vi "F-Zones.vi"(8 "Filter Prams In":T3, 10 "Trans Geometry (mm)":T1={"Transducer"=0, "Geo Focus"=12.0, "a (radius)"=3.0, "# of rings"=5, "kerf space "=0.1, "Center Freq"=12.0} {"Transducer" items=["6D 12R 40 MHz"=0, "10D 31R 20 MHz"=1, "10D 23R 20 MHz"=2, "6D 23R 40 MHz"=3, "4.5D 10.7R 40 MHz"=4, "9D 23.5R 20 MHz"=5, "9D 25.8R 20MHz"=6, "Enter"=99]}) -> (0 "Filter Prams":T3, 2 "ROC (m)":dbl, 3 "annuli rad (m)":dbl[](array[numeric]), 5 "Trans Geometry (mm) out":T1={"Transducer"=0, "Geo Focus"=12.0, "a (radius)"=3.0, "# of rings"=5, "kerf space "=0.1, "Center Freq"=12.0} {"Transducer" items=["6D 12R 40 MHz"=0, "10D 31R 20 MHz"=1, "10D 23R 20 MHz"=2, "6D 23R 40 MHz"=3, "4.5D 10.7R 40 MHz"=4, "9D 23.5R 20 MHz"=5, "9D 25.8R 20MHz"=6, "Enter"=99]})   [LabVIEW 2022 SP3]
uses:
  -AnnularRoutines/TransGeometry.ctl
  -AnnularRoutines/ArrayGeometry.ctl
panel:
  in  "Filter Prams 2":T3={"low cutoff"=5, "order"=81, "high cutoff"=35}
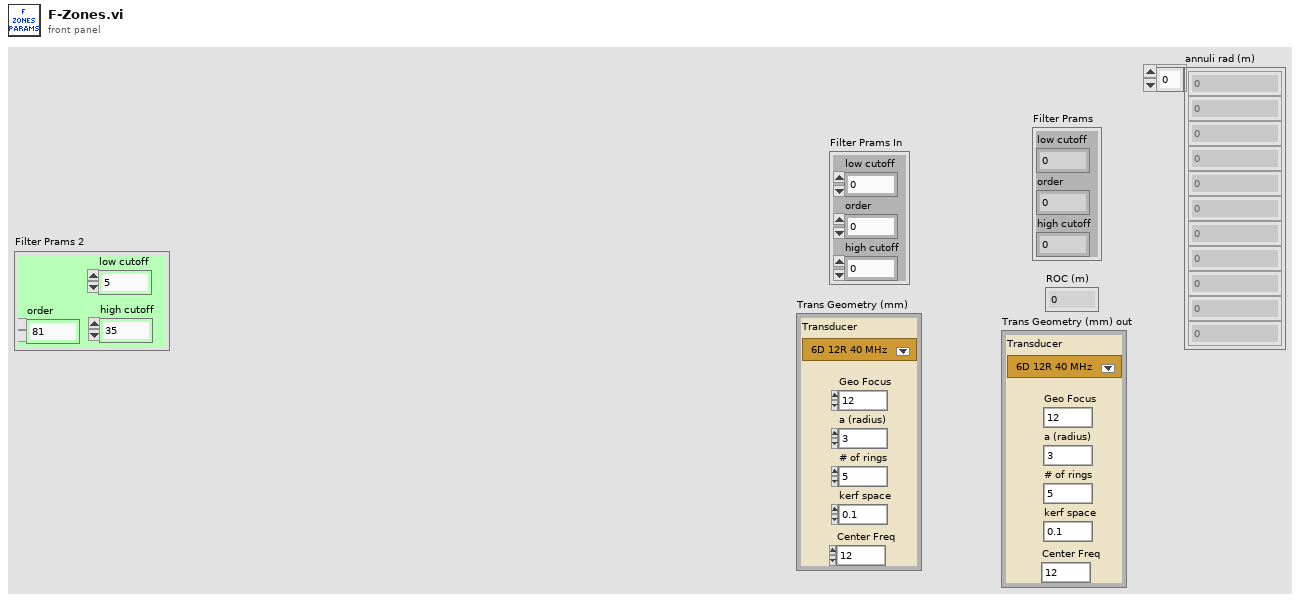
[diagram p1: front panel]
types:
  T1 = typedef "TransGeometry.ctl" = cluster{"Transducer":T2, "Geo Focus":dbl, "a (radius)":dbl, "# of rings":i32, "kerf space ":dbl, "Center Freq":dbl}
  T2 = typedef "ArrayGeometry.ctl" = u16
  T3 = cluster{"low cutoff":i32, "order":i32, "high cutoff":i32}
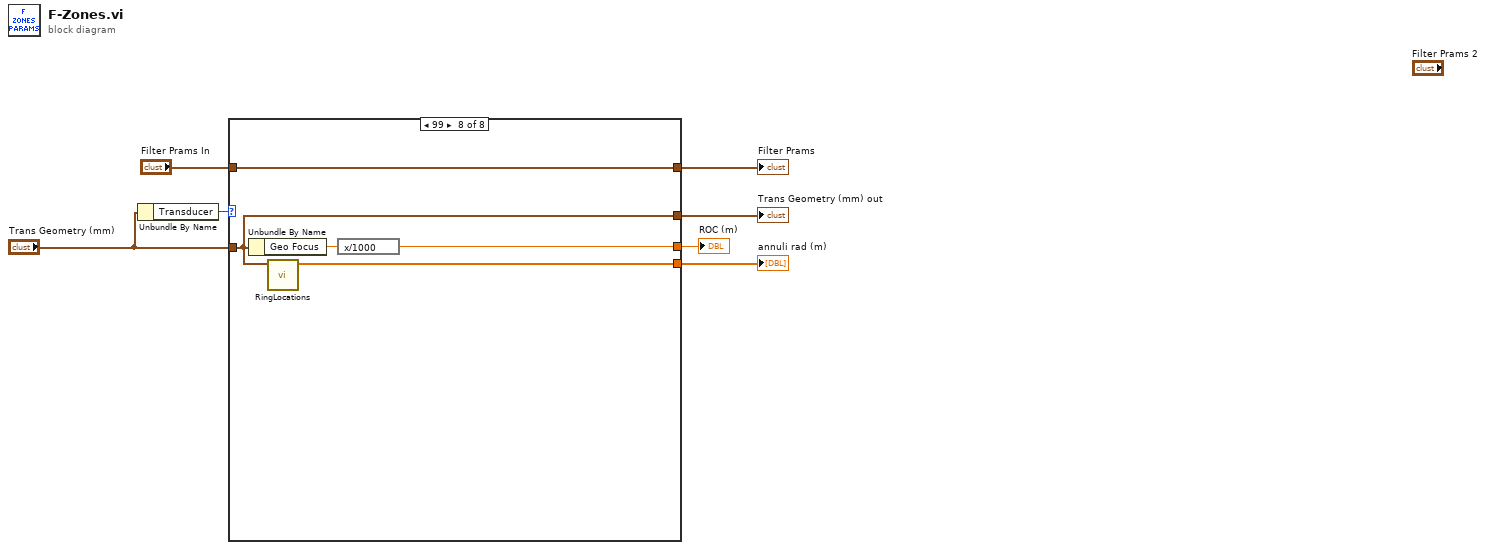
[diagram p0: block diagram]
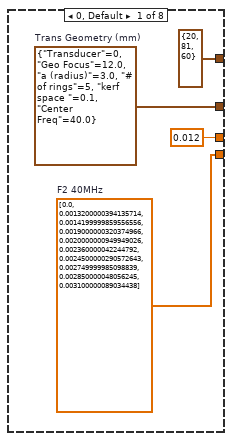
[diagram p2: hidden frame]
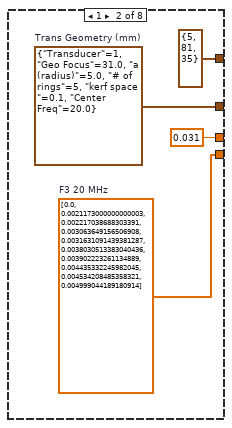
[diagram p3: hidden frame]
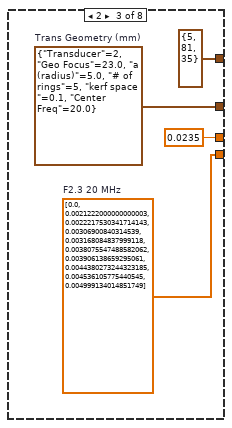
[diagram p4: hidden frame]
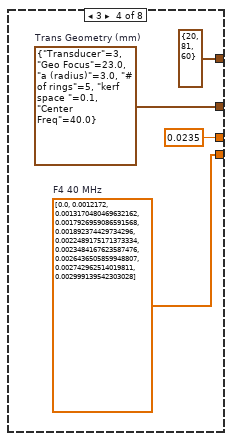
[diagram p5: hidden frame]
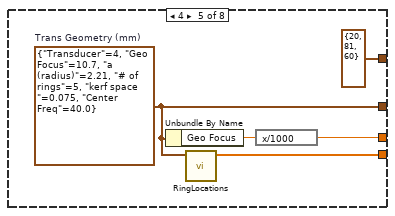
[diagram p6: hidden frame]
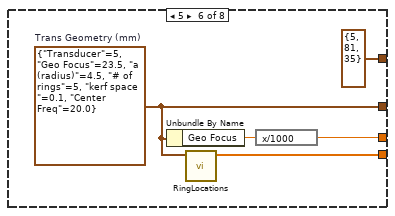
[diagram p7: hidden frame]
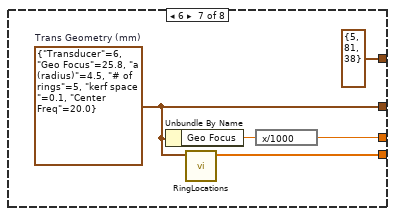
[diagram p8: hidden frame]
diagram:
  n1 = Unbundle By Name("Trans Geometry (mm)") -> ("Transducer"=w3:T2)
  n2 = case shown="99" w3 {
    tunnel: [w10 w14 w17 w21 w28 w33 w38 w43] -> w6
    tunnel: [0.012 ("ROC (mm)") 0.031 ("ROC (mm)") 0.0235 ("ROC (mm)") 0.0235 ("ROC (mm)") w26 w31 w36 w41] -> w7
    tunnel: [T3 {"low cutoff"=20, "order"=81, "high cutoff"=60} ("Filter Prams") T3 {"low cutoff"=5, "order"=81, "high cutoff"=35} ("Filter Prams") T3 {"low cutoff"=5, "order"=81, "high cutoff"=35} ("Filter Prams") T3 {"low cutoff"=20, "order"=81, "high cutoff"=60} ("Filter Prams") T3 {"low cutoff"=20, "order"=81, "high cutoff"=60} ("Filter Prams") T3 {"low cutoff"=5, "order"=81, "high cutoff"=35} ("Filter Prams") T3 {"low cutoff"=5, "order"=81, "high cutoff"=38} ("Filter Prams") w40] -> w5
    tunnel: "Filter Prams In" -> [_ _ _ _ _ _ _ w40]
    tunnel: "Trans Geometry (mm)" -> [_ _ _ _ _ _ _ w39]
    tunnel: [w8 w12 w16 w20 w24 w29 w34 w39] -> w1
    frame 0, Default {
      w8 = T1 {"Transducer"=0, "Geo Focus"=12.0, "a (radius)"=3.0, "# of rings"=5, "kerf space "=0.1, "Center Freq"=40.0}  # Trans Geometry (mm)
      w10 = sgl[] [0.0, 0.00132, 0.00142, 0.0019, 0.002, 0.00236, 0.00245, 0.00275, 0.00285, 0.0031]  # F2 40MHz
    }
    frame 1 {
      w12 = T1 {"Transducer"=1, "Geo Focus"=31.0, "a (radius)"=5.0, "# of rings"=5, "kerf space "=0.1, "Center Freq"=20.0}  # Trans Geometry (mm)
      w14 = dbl[] [0.0, 0.0021173000000000003, 0.002217038688303391, 0.003063649156506908, 0.0031631091439381287, 0.0038030513383040436, 0.003902223261134889, 0.004435332245982045, 0.004534208485358321, 0.004999044189180914]  # F3 20 MHz
    }
    frame 2 {
      w16 = T1 {"Transducer"=2, "Geo Focus"=23.0, "a (radius)"=5.0, "# of rings"=5, "kerf space "=0.1, "Center Freq"=20.0}  # Trans Geometry (mm)
      w17 = dbl[] [0.0, 0.0021222000000000003, 0.0022217530341714143, 0.00306900840314539, 0.003168084837999118, 0.0038075547488582062, 0.003906138659295061, 0.0044380273244323185, 0.004536105775440545, 0.004999134014851749]  # F2.3 20 MHz
    }
    frame 3 {
      w20 = T1 {"Transducer"=3, "Geo Focus"=23.0, "a (radius)"=3.0, "# of rings"=5, "kerf space "=0.1, "Center Freq"=40.0}  # Trans Geometry (mm)
      w21 = dbl[] [0.0, 0.0012172, 0.0013170480469632162, 0.0017926959086591568, 0.001892374429734296, 0.0022489175171373334, 0.0023484167623587476, 0.0026436505859948807, 0.002742962514019811, 0.002999139542303028]  # F4 40 MHz
    }
    frame 4 {
      w24 = T1 {"Transducer"=4, "Geo Focus"=10.7, "a (radius)"=2.21, "# of rings"=5, "kerf space "=0.075, "Center Freq"=40.0}  # Trans Geometry (mm)
      n3 = Unbundle By Name(w24) -> ("Geo Focus"=w27:dbl)
      n4 = call "RingLocations.vi"("Trans Geometry (mm)"=w24) -> ("rings (m)"=w28:dbl[])  [unwired: 9 in, 1 out]
      n5 = expression code="x/1000"(w27) -> (w26:dbl)
    }
    frame 5 {
      w29 = T1 {"Transducer"=5, "Geo Focus"=23.5, "a (radius)"=4.5, "# of rings"=5, "kerf space "=0.1, "Center Freq"=20.0}  # Trans Geometry (mm)
      n6 = Unbundle By Name(w29) -> ("Geo Focus"=w32:dbl)
      n7 = call "RingLocations.vi"("Trans Geometry (mm)"=w29) -> ("rings (m)"=w33:dbl[])  [unwired: 9 in, 1 out]
      n8 = expression code="x/1000"(w32) -> (w31:dbl)
    }
    frame 6 {
      w34 = T1 {"Transducer"=6, "Geo Focus"=25.8, "a (radius)"=4.5, "# of rings"=5, "kerf space "=0.1, "Center Freq"=20.0}  # Trans Geometry (mm)
      n9 = Unbundle By Name(w34) -> ("Geo Focus"=w37:dbl)
      n10 = call "RingLocations.vi"("Trans Geometry (mm)"=w34) -> ("rings (m)"=w38:dbl[])  [unwired: 9 in, 1 out]
      n11 = expression code="x/1000"(w37) -> (w36:dbl)
    }
    frame 99 {
      n12 = Unbundle By Name(w39) -> ("Geo Focus"=w42:dbl)
      n13 = call "RingLocations.vi"("Trans Geometry (mm)"=w39) -> ("rings (m)"=w43:dbl[])  [unwired: 9 in, 1 out]
      n14 = expression code="x/1000"(w42) -> (w41:dbl)
    }
  }
  "ROC (m)" <- w7
  "annuli rad (m)" <- w6
  "Filter Prams" <- w5
  "Trans Geometry (mm) out" <- w1
